vi "Focusing.vi"(9 "Filter Type":T2(ring)=enum."Differentiation", 11 "Image Path":path=path "D:/Inward_Lens_Tuning/Sample Images/img_34.jpeg") -> (0 "error out":errorcluster, 1 "Curent Mean Value":sgl=4.1535125 format="%.2f", 2 "Mean Value Max":sgl=4.1535125 format="%.2f", 3 "Pattern Presence":bool=TRUE, 5 "Image out":T1(plugin-control))   [LabVIEW 2019]
uses:
  <vilib>/vision/NI_Vision_Development_Module.lvlib
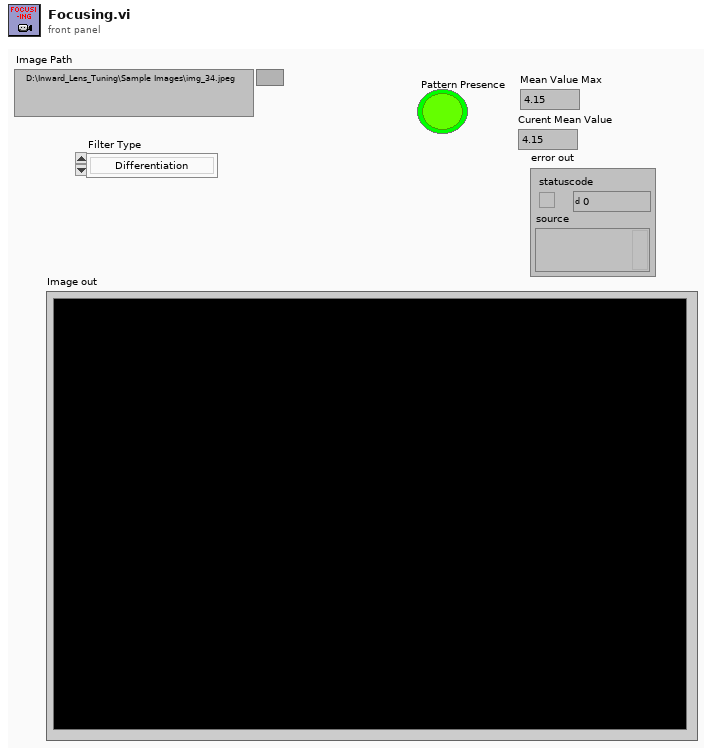
[diagram p1: front panel]
types:
  T1 = typedef "IMAQ Image.ctl" = refnum<image>
  T2 = enum16{"Convolution", "Differentiation", "Gradient", "Prewitt", "Roberts", "Sigma", "Sobel"}
  T3 = typedef "Image Type" = u32
  T4 = enum32{"Differentiation", "Gradient", "Prewitt", "Roberts", "Sigma", "Sobel"}
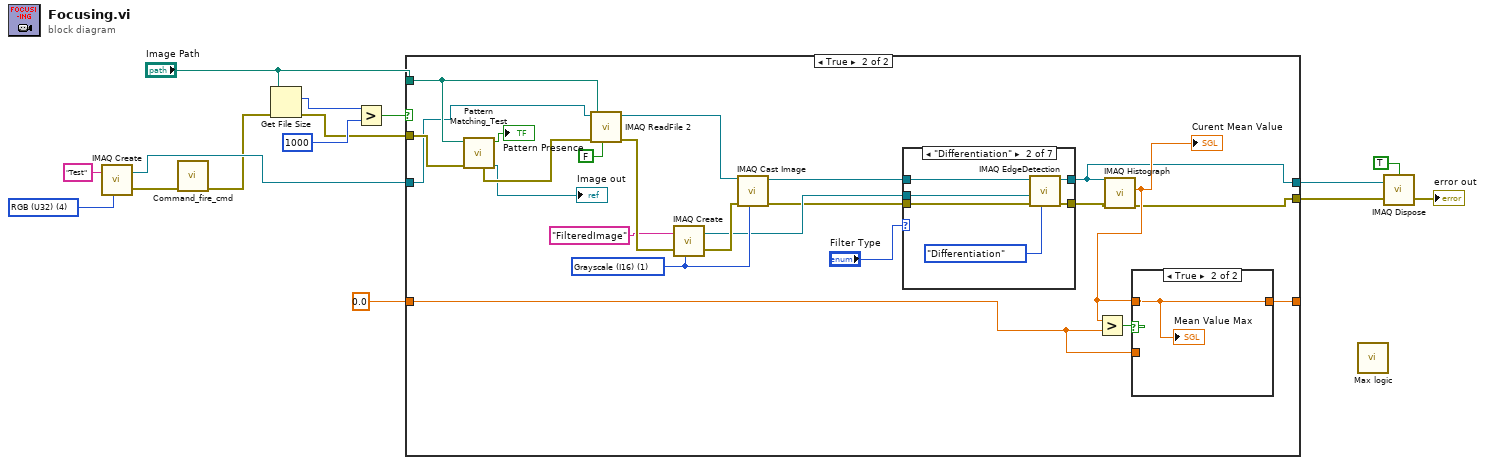
[diagram p0: block diagram]
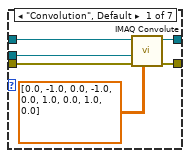
[diagram p4: hidden frame]
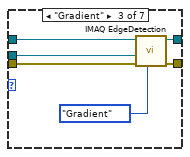
[diagram p5: hidden frame]
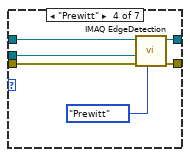
[diagram p6: hidden frame]
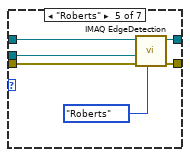
[diagram p7: hidden frame]
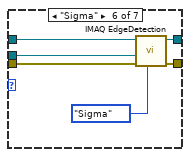
[diagram p8: hidden frame]
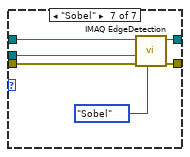
[diagram p9: hidden frame]
diagram:
  w9 = T3 4 items=["Grayscale (U8)", "Grayscale (I16)", "Grayscale (SGL)", "Complex (CSG)", "RGB (U32)", "HSL (U32)", "RGB (U64)", "Grayscale (U16)"] ("Image Type")
  n1 = call "IMAQ Create"("Image Name"="Test", "Image Type"=w9) -> ("New Image"=w3:T1, "error out"=w4:errorcluster)  [unwired: 3 in]
  n2 = call "Command_fire_cmd.vi"("error in"=w4) -> ("error out"=w2:errorcluster)  [unwired: 6 in, 2 out]
  n3 = Get File Size(file="Image Path", error in=w2) -> (size (in bytes)=w7:i64, 0:w1:errorcluster)  [unwired: 1 out]
  n4 = Greater?(x=w7, y=i64 1000) -> (0:w5:bool)
  n5 = case shown="True" w5 {
    tunnel: "Image Path" -> [_ w40]
    tunnel: w1 -> [w17 w39]
    tunnel: [w18 w26] -> _
    tunnel: 0.0 -> [w18 w21]
    tunnel: w3 -> [w16 w25]
    tunnel: [w17 w23] -> w14
    tunnel: [w16 w22] -> w13
    frame False {
    }
    frame True {
      w33 = T3 1 items=["Grayscale (U8)", "Grayscale (I16)", "Grayscale (SGL)", "Complex (CSG)", "RGB (U32)", "HSL (U32)", "RGB (U64)", "Grayscale (U16)"] ("Image Type")
      n6 = call "Pattern Matching_Test.vi"("error in (no error)"=w39, "File Path"=w40) -> ("Image out"=→"Image out":T1, "Pattern Presence"=→"Pattern Presence":bool, "error out"=w38:errorcluster)  [unwired: 5 in, 2 out]
      n7 = call "IMAQ ReadFile 2"("Use File Path Image Type"=FALSE, "File Path"=w40, "error in (no error)"=w38, "Image"=w25) -> ("error out"=w36:errorcluster, "Image Out"=w20:T1)  [unwired: 3 in, 3 out]
      n8 = call "IMAQ Create"("Image Name"="FilteredImage", "Image Type"=w33, "error in (no error)"=w36) -> ("New Image"=w30:T1, "error out"=w34:errorcluster)  [unwired: 2 in]
      n9 = call "IMAQ Cast Image"("Image Type"=w33, "error in (no error)"=w34, "Image Src"=w20) -> ("error out"=w29:errorcluster, "Image Dst Out"=w31:T1)  [unwired: 7 in]
      n10 = case shown="\"Differentiation\"" "Filter Type" {
        tunnel: w31 -> [w48 w54 w60 w66 w72 w78 w84]
        tunnel: w29 -> [w47 w53 w59 w65 w71 w77 w83]
        tunnel: w30 -> [w46 w55 w61 w67 w73 w79 w85]
        tunnel: [w45 w50 w56 w62 w68 w74 w80] -> w28
        tunnel: [w44 w51 w57 w63 w69 w75 w81] -> w22
        frame "Convolution", Default {
          n11 = call "IMAQ Convolute"("Kernel"=sgl[][] [[0.0, -1.0, 0.0], [-1.0, 0.0, 1.0], [0.0, 1.0, 0.0]], "error in (no error)"=w47, "Image Dst"=w46, "Image Src"=w48) -> ("error out"=w45:errorcluster, "Image Dst Out"=w44:T1)  [unwired: 6 in]
        }
        frame "Differentiation" {
          n12 = call "IMAQ EdgeDetection"("Method"=T4."Differentiation", "error in (no error)"=w53, "Image Dst"=w55, "Image Src"=w54) -> ("error out"=w50:errorcluster, "Image Dst Out"=w51:T1)  [unwired: 6 in]
        }
        frame "Gradient" {
          n13 = call "IMAQ EdgeDetection"("Method"=T4."Gradient", "error in (no error)"=w59, "Image Dst"=w61, "Image Src"=w60) -> ("error out"=w56:errorcluster, "Image Dst Out"=w57:T1)  [unwired: 6 in]
        }
        frame "Prewitt" {
          n14 = call "IMAQ EdgeDetection"("Method"=T4."Prewitt", "error in (no error)"=w65, "Image Dst"=w67, "Image Src"=w66) -> ("error out"=w62:errorcluster, "Image Dst Out"=w63:T1)  [unwired: 6 in]
        }
        frame "Roberts" {
          n15 = call "IMAQ EdgeDetection"("Method"=T4."Roberts", "error in (no error)"=w71, "Image Dst"=w73, "Image Src"=w72) -> ("error out"=w68:errorcluster, "Image Dst Out"=w69:T1)  [unwired: 6 in]
        }
        frame "Sigma" {
          n16 = call "IMAQ EdgeDetection"("Method"=T4."Sigma", "error in (no error)"=w77, "Image Dst"=w79, "Image Src"=w78) -> ("error out"=w74:errorcluster, "Image Dst Out"=w75:T1)  [unwired: 6 in]
        }
        frame "Sobel" {
          n17 = call "IMAQ EdgeDetection"("Method"=T4."Sobel", "error in (no error)"=w83, "Image Dst"=w85, "Image Src"=w84) -> ("error out"=w80:errorcluster, "Image Dst Out"=w81:T1)  [unwired: 6 in]
        }
      }
      n18 = call "IMAQ Histograph"("error in (no error)"=w28, "Image"=w22) -> ("error out"=w23:errorcluster, "Mean Value"=w24:sgl)  [unwired: 6 in, 2 out]
      "Curent Mean Value" <- w24
      n19 = Greater?(x=w24, y=w21) -> (0:w27:bool)
      n20 = case shown="True" w27 {
        tunnel: w24 -> [_ w43]
        tunnel: [w42 w43] -> w26
        tunnel: w21 -> [w42 _]
        frame False {
        }
        frame True {
          "Mean Value Max" <- w43
        }
      }
    }
  }
  n21 = call "Max logic.vi"() -> ()  [unwired: 12 in]
  n22 = call "IMAQ Dispose"("All Images? (No)"=TRUE, "Image"=w13, "error in (no error)"=w14) -> ("error out"=→"error out":errorcluster)  [unwired: 3 in]
